vi "LOGtree.vi"   [LabVIEW 2025, in "LOGlib.lvlib"]
uses:
  LOGlib.lvlib
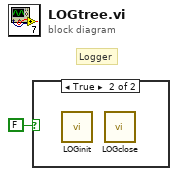
[diagram p0: block diagram]
diagram:
  # "Logger"
  n1 = case shown="True" FALSE {
    frame False {
    }
    frame True {
      n2 = call "LOGinit.vi"() -> ()  [unwired: 11 in, 1 out]
      n3 = call "LOGclose.vi"() -> ()  [unwired: 12 in]
    }
  }
